vi "SlewRateLimiter_Reset.vi"(8 "Time":dbl=-1.0 format="%33.4f", 9 "ResetValue":dbl, 11 "in SLEW_RATE_LIMITER":T1 {"PrevTime" format="%30.5p"; "PrevValue" format="%13.5p"; "RateLimit" format="%13.5p"}) -> (3 "out SLEW_RATE_LIMITER":T1 {"PrevTime" format="%30.5p"; "PrevValue" format="%13.5p"; "RateLimit" format="%13.5p"})   [LabVIEW 2019, in "Trajectory_Library.lvlib"]
doc: "Resets the slew rate limiter to the specified value; ignores the rate limit when doing so.\n \nInputs: \n - in Slew Rate Limiter -- The Slew Rate Limiter data cluster\n - ResetValue -- The value to reset to.\n \n \nOutputs:\n - out Slew Rate Limiter -- The modified Slew Rate Limiter data cluster"
uses:
  Trajectory_Library.lvlib
  TypeDef/SLEW_RATE_LIMITER.ctl
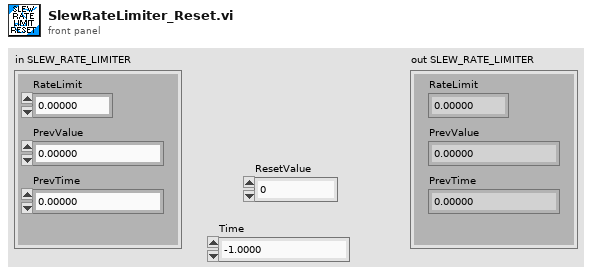
[diagram p1: front panel]
types:
  T1 = typedef "Trajectory_Library.lvlib/SLEW_RATE_LIMITER.ctl" = cluster{"RateLimit":dbl, "PrevValue":dbl, "PrevTime":dbl}
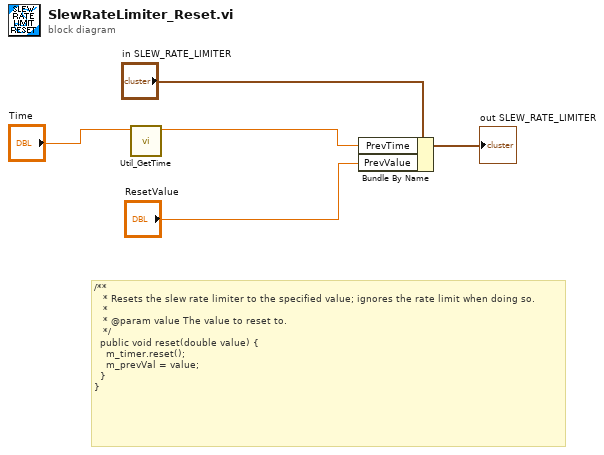
[diagram p0: block diagram]
diagram:
  # "/**\n   * Resets the slew rate limiter to the specified value; ignores the rate limit when doing so.\n   *\n   * @param value The value to reset to.\n   */\n  public void reset(double value) {\n    m_timer.reset();\n    m_prevVal = value;\n  }\n}"
  n1 = call "Util_GetTime.vi"("Pass_Through_Time"="Time") -> ("FPGA_Time_Seconds"=w2:dbl)  [unwired: 9 in, 1 out]
  n2 = Bundle By Name(cluster="in SLEW_RATE_LIMITER", "PrevTime"=w2, "PrevValue"="ResetValue") -> (→"out SLEW_RATE_LIMITER":T1)
